vi "Position_Update.vi"(11 "Field_Drive":T2) -> (3 "Field_Drive_Out":T1)   [LabVIEW 2012]
uses:
  Field_Drive_in.ctl
  Field_Drive_out.ctl
  C:/Program Files (x86)/National Instruments/LabVIEW 2012/examples/FRC/I2C/ADXL345 I2C/Driver/ADXL345 I2C Axis.ctl
  <vilib>/ptbypt/NI_PtbyPt.lvlib
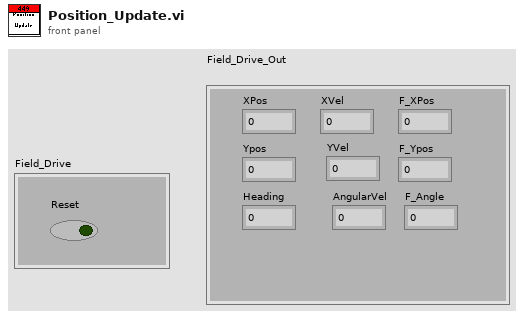
[diagram p1: front panel]
types:
  T1 = typedef "Field_Drive_out.ctl" = cluster{"XPos":dbl, "Ypos":dbl, "XVel":dbl, "YVel":dbl, "Heading":dbl, "AngularVel":dbl, "F_XPos":dbl, "F_Ypos":dbl, "F_Angle":dbl}
  T2 = typedef "Field_Drive_in.ctl" = cluster{"Reset":bool}
  T3 = typedef "ADXL345 I2C Axis.ctl" = u8
  T4 = typedef "WPI_I2CDevRef.ctl" = cluster{"DevStatus":errorcluster, "Digital Module":T5, "Device Address":u8}
  T5 = typedef "FPGA_TypedefDigitalModule.ctl" = enum16{"Digital Module 1", "Digital Module 2"}
  T6 = typedef "WPI_GyroDevRef.ctl" = cluster{"DevStatus":errorcluster, "Analog Module":T7, "Analog Channel":T8, "Offset":dbl, "Gain (VoltsPerDegree/Second)":dbl}
  T7 = typedef "FPGA_TypedefAnalogModule.ctl" = enum16{"Analog Module 1", "Analog Module 2"}
  T8 = typedef "FPGA_AIChannel.ctl" = enum8{"AI 1", "AI 2", "AI 3", "AI 4", "AI 5", "AI 6", "AI 7", "AI 8", "Invalid"}
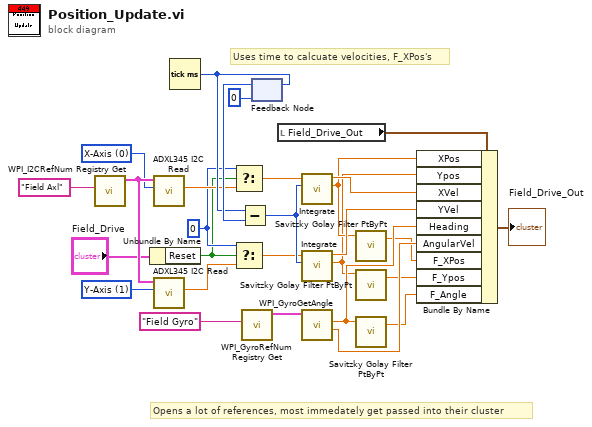
[diagram p0: block diagram]
diagram:
  w16 = 0
  w23 = T3 1 items=["X-Axis", "Y-Axis", "Z-Axis"] ("Axis")
  w24 = T3 0 items=["X-Axis", "Y-Axis", "Z-Axis"] ("Axis")
  # "Uses time to calcuate velocities, F_XPos's"
  # "Opens a lot of references, most immedately get passed into their cluster"
  n1 = call <vilib>:"WPI_I2CRefNum Registry Get.vi"("refnum name"="Field Axl") -> ("I2CDevRef"=w25:T4)  [unwired: 9 in, 1 out]
  n2 = Unbundle By Name("Field_Drive") -> ("Reset"=w12:bool)
  n3 = call "ADXL345 I2C Read.vi"("Axis"=w24, "I2CDevRef"=w25) -> ("Acceleration"=w18:dbl)  [unwired: 7 in, 2 out]
  n4 = call "ADXL345 I2C Read.vi"("Axis"=w23, "I2CDevRef"=w25) -> ("Acceleration"=w17:dbl)  [unwired: 7 in, 2 out]
  n5 = Tick Count (ms)() -> (millisecond timer value=w20:u32)
  n6 = Select(t=w16, s=w12, f=w18) -> (s? t:f=w14:dbl)
  n7 = Select(t=w16, s=w12, f=w17) -> (s? t:f=w15:dbl)
  n8 = call <vilib>:"WPI_GyroRefNum Registry Get.vi"("refnum name"="Field Gyro") -> ("GyroDevRef"=w27:T6)  [unwired: 9 in, 1 out]
  n9 = feedback-in #1(w20) -> ()
  n10 = feedback #1(u32 0 ("millisecond timer value")) -> (w21:u32)
  n11 = Subtract(x=w20, y=w21) -> (x-y=w19:u32)
  n12 = local read "Field_Drive_Out"() -> (w11:T1)
  n13 = call "Integrate.vi"("dt"=w19, "Acceleration"=w14) -> ("Displacememt"=w2:dbl, "Velocity"=w9:dbl)  [unwired: 8 in]
  n14 = call "Integrate.vi"("dt"=w19, "Acceleration"=w15) -> ("Displacememt"=w1:dbl, "Velocity"=w8:dbl)  [unwired: 8 in]
  n15 = call <vilib>:"WPI_GyroGetAngle.vi"("GyroDevRef"=w27) -> ("Angular Rate"=w6:dbl, "Angle"=w7:dbl)  [unwired: 7 in, 2 out]
  n16 = call <vilib>:"Savitzky Golay Filter PtByPt.vi"("x"=w2) -> ("Filtered x"=w4:dbl)  [unwired: 3 in, 1 out]
  n17 = call <vilib>:"Savitzky Golay Filter PtByPt.vi"("x"=w1) -> ("Filtered x"=w3:dbl)  [unwired: 3 in, 1 out]
  n18 = call <vilib>:"Savitzky Golay Filter PtByPt.vi"("x"=w7) -> ("Filtered x"=w5:dbl)  [unwired: 3 in, 1 out]
  n19 = Bundle By Name(cluster=w11, "XPos"=w2, "Ypos"=w1, "XVel"=w9, "YVel"=w8, "Heading"=w7, "AngularVel"=w6, "F_XPos"=w4, "F_Ypos"=w3, "F_Angle"=w5) -> (→"Field_Drive_Out":T1)
